vi "get channels.vi"(8 "error in (no error)":errorcluster, 11 "Template Action Cfg in":refnum<class "Template Action Cfg.lvclass">) -> (0 "error out":errorcluster, 2 "action channels":refnum<class "TBM channel.lvclass">[](array[class]), 3 "Template Action Cfg out":refnum<class "Template Action Cfg.lvclass">)   [LabVIEW 2014, in "Template Action Cfg.lvclass"]
uses:
  Template Action Cfg.lvclass
  <vilib>/NI/Tag Bus Module Framework/channel/TBM channel.lvclass
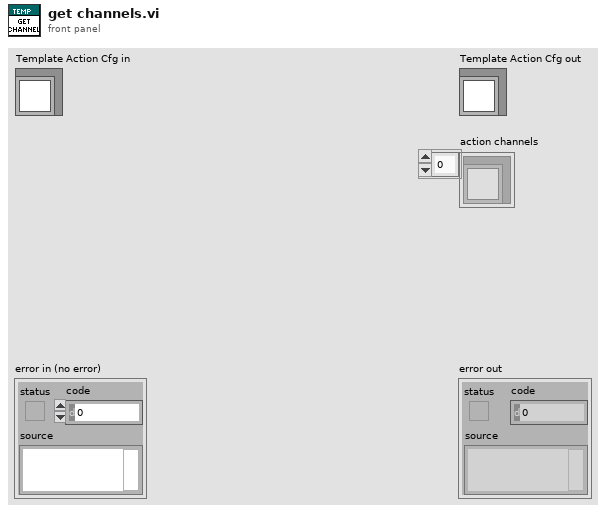
[diagram p1: front panel]
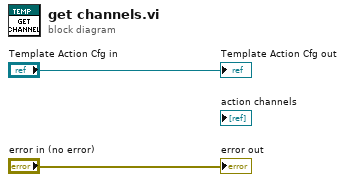
[diagram p0: block diagram]
diagram:
  "error out" <- "error in (no error)"
  "Template Action Cfg out" <- "Template Action Cfg in"
